vi "guid.vi"() -> (6 "name (unnamed)":string)   [LabVIEW 2018]
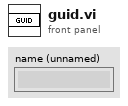
[diagram p1: front panel]
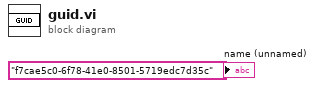
[diagram p0: block diagram]
diagram:
  "name (unnamed)" <- "f7cae5c0-6f78-41e0-8501-5719edc7d35c" ("name (unnamed)")
